vi "Heater_Setpoint_Names.vi"(2 "Reload from file":bool) -> (4 "Chs to Activate":string[](array[string]), 5 "Temp Chs":string[](array[string]), 6 "Setpoint Chs":string[](array[string]), 7 "Power Chs":string[](array[string]), 8 "Setpoint Values":dbl[](array[numeric]))   [LabVIEW 2010]
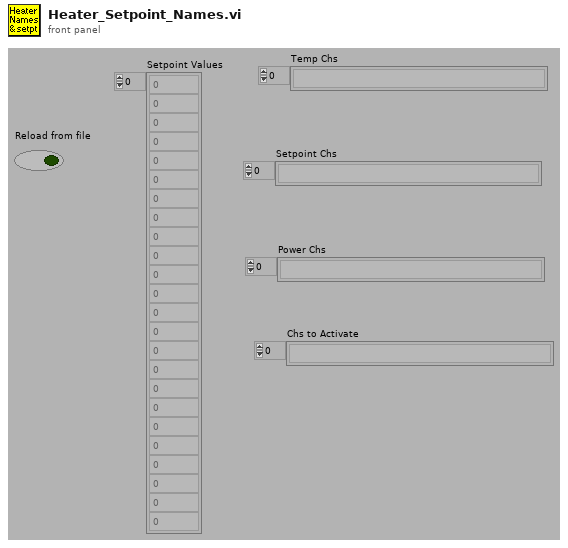
[diagram p1: front panel]
types:
  T1 = typedef "Heater_Setpoint.ctl" = cluster{"Ch Name":string, "Setpoint":dbl}
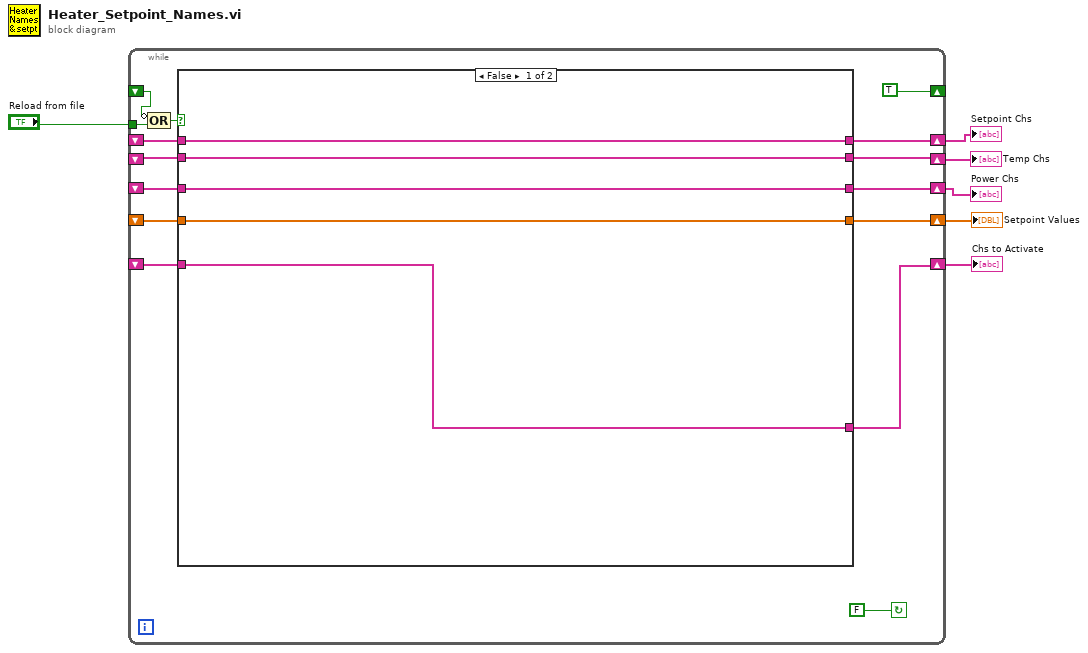
[diagram p0: block diagram]
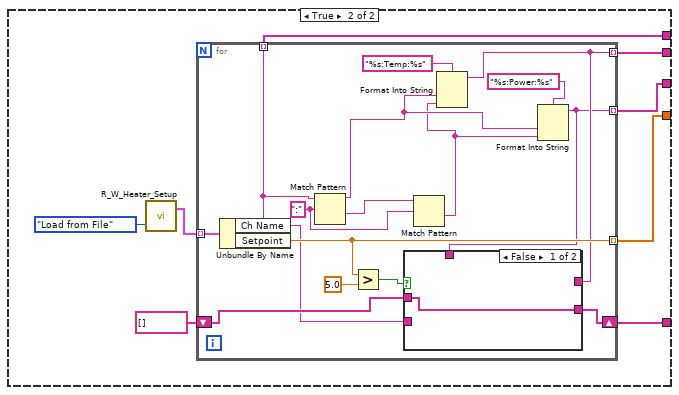
[diagram p2: hidden frame]
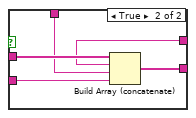
[diagram p3: hidden frame]
diagram:
  n1 = while {
    shift-left: _ -> [w16]
    shift-right: [TRUE] -> _
    shift-left: _ -> [w19]
    shift-right: [w21] -> w6
    tunnel: "Reload from file" -> [w17]
    shift-right: [w14] -> w4
    shift-left: _ -> [w13]
    shift-right: [w12] -> w3
    shift-left: _ -> [w11]
    shift-right: [w9] -> w2
    shift-left: _ -> [w10]
    shift-right: [w8] -> w1
    shift-left: _ -> [w7]
    stop <- FALSE continue-if-true
    n2 = Compound Arithmetic op=OR(invert w16, w17) -> (w15:bool)
    n3 = case shown="False" w15 {
      tunnel: [w26 w29] -> w21
      tunnel: w19 -> [w26 _]
      tunnel: [w25 w32] -> w14
      tunnel: w13 -> [w25 _]
      tunnel: [w24 w31] -> w12
      tunnel: w11 -> [w24 _]
      tunnel: w10 -> [w23 _]
      tunnel: [w23 w30] -> w9
      tunnel: [w22 w27] -> w8
      tunnel: w7 -> [w22 _]
      frame False {
      }
      frame True {
        n4 = call "R_W_Heater_Setup.vi"("Mode"=enum16{"Load from File", "Save to File"}."Load from File") -> ("Setpoints Out"=w33:T1[])  [unwired: 1 in, 1 out]
        n5 = for {
          tunnel: w33 -> [w49] mode=indexing
          tunnel: [w42] -> w32 mode=indexing
          tunnel: [w36] -> w31 mode=indexing
          tunnel: [w37] -> w30 mode=indexing
          tunnel: [w38] -> w29 mode=indexing
          shift-right: [w35] -> w27
          shift-left: string[] [] -> [w39]
          w47 = ":" ("regular expression")
          n6 = Unbundle By Name(w49) -> ("Ch Name"=w36:string, "Setpoint"=w42:dbl)
          n7 = Match Pattern(string=w36, regular expression=w47) -> (before substring=w44:string, after substring=w48:string)  [unwired: 3 out]
          n8 = Greater?(x=w42, y=5.0) -> (0:w40:bool)
          n9 = Match Pattern(string=w48, regular expression=w47) -> (after substring=w43:string)  [unwired: 4 out]
          n10 = Format Into String(format string="%s:Temp:%s", w44, w43) -> (resulting string=w38:string)  [unwired: 2 in, 1 out]
          n11 = Format Into String(format string="%s:Power:%s", w44, w43) -> (resulting string=w37:string)  [unwired: 2 in, 1 out]
          n12 = case shown="False" w40 {
            tunnel: w39 -> [w50 w55]
            tunnel: w38 -> [_ w54]
            tunnel: w37 -> [_ w53]
            tunnel: w36 -> [_ w52]
            tunnel: [w50 w51] -> w35
            frame False {
            }
            frame True {
              n13 = Build Array (concatenate)(w55, w54, w53, w52) -> (w51:string[])
            }
          }
        }
      }
    }
  }
  "Temp Chs" <- w6
  "Setpoint Values" <- w4
  "Setpoint Chs" <- w3
  "Power Chs" <- w2
  "Chs to Activate" <- w1
